vi "Cut from start of datum.vi"(2 "length":i32, 3 "datum":T1) -> (0 "data":u8[](array[numeric]) format="%02x", 1 "datum out":T1)   [LabVIEW 2020, in "NI_Bytestream.lvlib" / "Bytestream.lvclass"]
uses:
  <vilib>/Array/Bytestream/Bytestream.lvclass
  <vilib>/Array/Bytestream/Datum.ctl
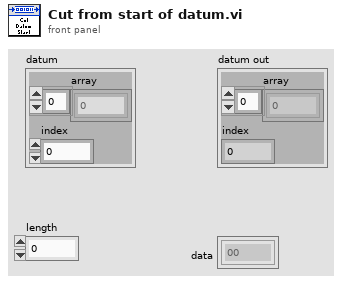
[diagram p1: front panel]
types:
  T1 = typedef "NI_Bytestream.lvlib/Bytestream.lvclass/Datum.ctl" = cluster{"array":u8[], "index":i32}
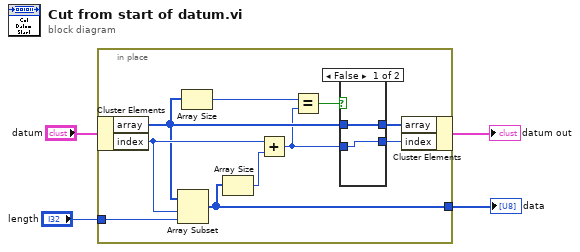
[diagram p0: block diagram]
diagram:
  n1 = in-place {
    in-place-border: "length" -> [w12]
    in-place-border: [w11] -> w1
    n2 = in-place-cluster #1("datum") -> ("array"=w8:u8[], "index"=w14:i32)
    n3 = Array Subset(array=w8, index=w14, length=w12) -> (w11:u8[])
    n4 = Array Size(array=w8) -> (size(s)=w13:i32)
    n5 = Array Size(array=w11) -> (size(s)=w10:i32)
    n6 = Add(x=w14, y=w10) -> (x+y=w7:i32)
    n7 = Equal?(x=w13, y=w7) -> (x = y?=w9:bool)
    n8 = case shown="False" w9 {
      tunnel: w8 -> [w16 _]
      tunnel: w7 -> [w15 _]
      tunnel: [w16 _] -> w6
      tunnel: [w15 _] -> w5
      frame False {
      }
      frame True {
      }
    }
    n9 = in-place-cluster #1("array"=w6, "index"=w5) -> (→"datum out":T1)
  }
  "data" <- w1
